vi "RSZVB Get Noise Figure Calibration State.vi"(8 "error in (no error)":errorcluster {"code" format="%.0x"}, 10 "Channel (1)":i32=1, 11 "VISA session":refnum<visa-resource-name>) -> (0 "error out":errorcluster {"code" format="%.0x"}, 1 "Calibration":bool, 3 "dup VISA session":refnum<visa-resource-name>)   [LabVIEW 2011]
doc: "This VI returns the state of the Noise Figure Calibration for the active channel <Ch>. \n\nNote(s):\n\n(1) This VI is available only with option R&S ZVAB-K30.\n\nRemote-control command(s):\n[SENSe<Ch>:]CORRection:NFIGure[:STATe]?"
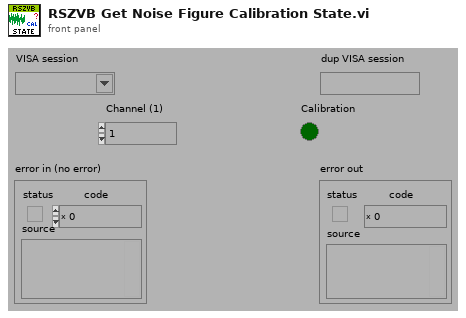
[diagram p1: front panel]
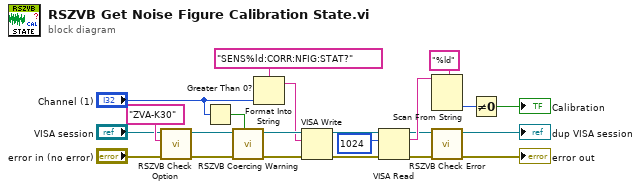
[diagram p0: block diagram]
diagram:
  n1 = call "RSZVB Check Option.vi"("error in (no error)"="error in (no error)", "Options"="ZVA-K30", "VISA session"="VISA session") -> ("error out"=w22:errorcluster, "dup VISA session"=w21:refnum<visa-resource-name>)  [unwired: 7 in]
  n2 = Greater Than 0?(x="Channel (1)") -> (x > 0?=w17:bool)
  n3 = call "RSZVB Coercing Warning.vi"("In Range?"=w17, "error in (no error)"=w22, "VISA session"=w21) -> ("error out"=w18:errorcluster, "dup VISA session"=w19:refnum<visa-resource-name>)  [unwired: 7 in]
  n4 = Format Into String(format string="SENS%ld:CORR:NFIG:STAT?", "Channel (1)") -> (resulting string=w16:string)  [unwired: 2 in, 1 out]
  n5 = VISA Write(VISA resource name=w19, write buffer=w16, error in (no error)=w18) -> (VISA resource name out=w7:refnum<visa-resource-name>, error out=w8:errorcluster)  [unwired: 1 out]
  n6 = VISA Read(VISA resource name=w7, byte count=u32 1024 ("byte count (0)"), error in (no error)=w8) -> (VISA resource name out=w10:refnum<visa-resource-name>, read buffer=w14:string, error out=w9:errorcluster)  [unwired: 1 out]
  n7 = Scan From String(format string="%ld", input string=w14) -> (output 1=w13:i32)  [unwired: 3 in, 3 out]
  n8 = call "RSZVB Check Error.vi"("error in (no error)"=w9, "VISA session"=w10) -> ("error out"=→"error out":errorcluster, "dup VISA session"=→"dup VISA session":refnum<visa-resource-name>)  [unwired: 8 in]
  n9 = Not Equal To 0?(x=w13) -> (x != 0?=→"Calibration":bool)
